vi "Ex2a gripper.vi"() -> ()   [LabVIEW 2013]
uses:
  ROS/Code/SubVIs/BaxterSide.ctl
panel:
  in  "Send":bool
  in  "% open":sgl=100.0 min=0 max=100
  in  "stop":bool
  in  "Side":T1=enum."right"
  # "Hit run to close and open the gripper"
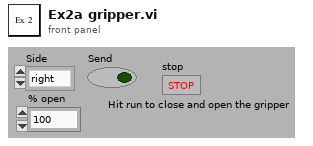
[diagram p1: front panel]
types:
  T1 = typedef "BaxterSide.ctl" = enum16{"left", "right"}
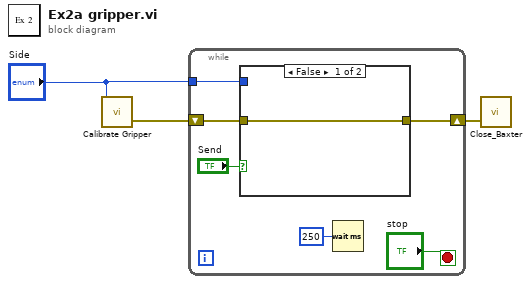
[diagram p0: block diagram]
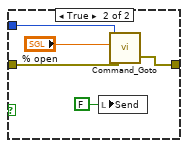
[diagram p2: hidden frame]
diagram:
  n1 = call "Calibrate Gripper.vi"("Side"="Side") -> ("error out"=w2:errorcluster)  [unwired: 5 in]
  n2 = while {
    tunnel: "Side" -> [w9]
    shift-right: [w6] -> w1
    shift-left: w2 -> [w8]
    stop <- "stop" stop-if-true
    n3 = case shown="False" "Send" {
      tunnel: w9 -> [_ w15]
      tunnel: w8 -> [w10 w14]
      tunnel: [w10 w13] -> w6
      frame False {
      }
      frame True {
        n4 = local write "Send"(FALSE ("Send")) -> ()
        n5 = call "Command_Goto.vi"("Side"=w15, "Desired Position"="% open", "error in"=w14) -> ("error out"=w13:errorcluster)  [unwired: 3 in]
      }
    }
    n6 = Wait (ms)(milliseconds to wait=u32 250) -> ()  [unwired: 1 out]
  }
  n7 = call "Close_Baxter.vi"("error in"=w1) -> ()  [unwired: 3 in, 1 out]
